vi "ScanIfSufficientPlaceHostDMA.vi"(8 "error in (no error)":errorcluster, 9 "Samples per Write":u32=1024000 format="%.3p", 10 "HSS Resource reference":refnum<k20>, 11 "TDMS controls in":T1[](array[typedef])) -> (0 "error out":errorcluster, 1 "Enough Space":bool, 2 "HSS Resource reference out":refnum<k20>, 3 "TDMS controls out":T1[](array[typedef]))   [LabVIEW 2018]
uses:
  TypeDefs/TDMS read.ctl
  <vilib>/Utility/error.llb/Error Cluster From Error Code.vi
  <vilib>/rvi/errors/niLvFpgaAdjustHostInterfaceError.vi
  <vilib>/rvi/interface/nirviMethod/nirviMethod.xnode
  <vilib>/FPGAPlugInAG/Dynamic/niLvFpga_AcquireWriteRegionFifo_Dynamic.vi
  <vilib>/rvi/errors/niLvFpgaMergeErrorWithErrorCode.vi
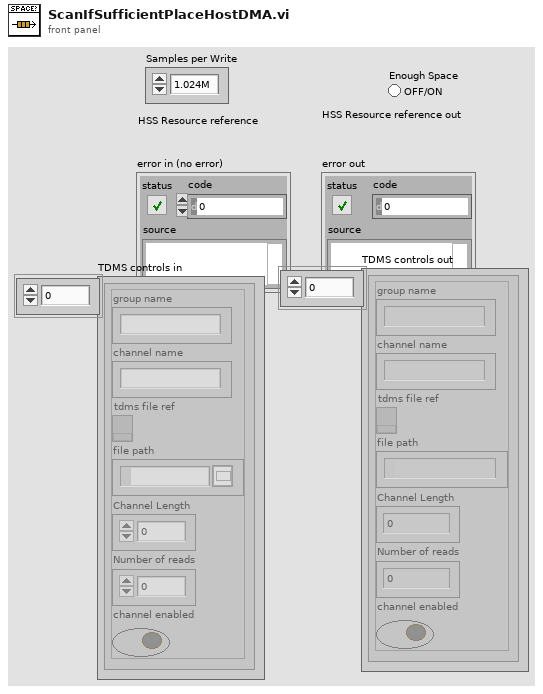
[diagram p1: front panel]
types:
  T1 = typedef "TDMS read.ctl" = cluster{"group name":string, "channel name":string, "tdms file ref":refnum<k34>, "file path":path, "Channel Length":i64, "Number of reads":i64, "channel enabled":bool}
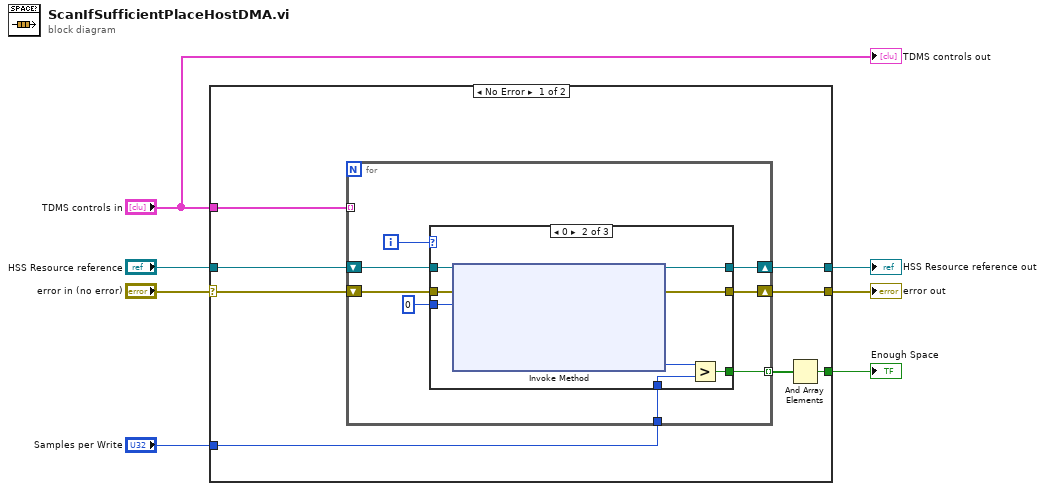
[diagram p0: block diagram]
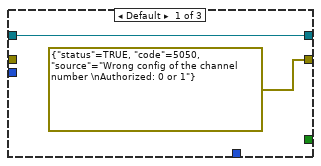
[diagram p2: hidden frame]
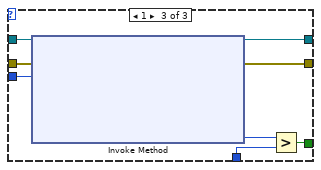
[diagram p3: hidden frame]
diagram:
  n1 = case shown="No Error" "error in (no error)" {
    selector: "error in (no error)" -> [w14 w43]
    tunnel: [w15 w43] -> w7
    tunnel: "Samples per Write" -> [w13 _]
    tunnel: [w11 _] -> w4
    tunnel: "HSS Resource reference" -> [w10 w42]
    tunnel: [w9 w42] -> w2
    tunnel: "TDMS controls in" -> [w8 _]
    frame No Error {
      n2 = for {
        shift-right: [w23] -> w15
        shift-left: w14 -> [w22]
        shift-right: [w21] -> w9
        shift-left: w10 -> [w20]
        tunnel: w13 -> [w18]
        tunnel: [w17] -> w12 mode=indexing
        tunnel: w8 -> [_] mode=indexing
        i -> [w16]
        n3 = case shown="0" w16 {
          tunnel: [errorcluster {"status"=TRUE, "code"=5050, "source"="Wrong config of the channel number \nAuthorized: 0 or 1"} ("error constant") w33 w41] -> w23
          tunnel: w22 -> [_ w32 w40]
          tunnel: [w25 w31 w39] -> w21
          tunnel: w20 -> [w25 w30 w38]
          tunnel: u32 0 ("Number of Elements") -> [_ w29 w37]
          tunnel: w18 -> [_ w27 w35]
          tunnel: [_ w26 w34] -> w17
          frame Default {
          }
          frame 0 {
            n4 = xnode "Invoke Method"("FPGA VI Reference In"=w30, "error in"=w32, "Number of Elements"=w29) -> ("FPGA VI Reference Out"=w31:refnum<k20>, "error out"=w33:errorcluster, "Empty Elements Remaining"=w28:u32)  [unwired: 1 in, 2 out]
            n5 = Greater?(x=w28, y=w27) -> (0:w26:bool)
          }
          frame 1 {
            n6 = xnode "Invoke Method"("FPGA VI Reference In"=w38, "error in"=w40, "Number of Elements"=w37) -> ("FPGA VI Reference Out"=w39:refnum<k20>, "error out"=w41:errorcluster, "Empty Elements Remaining"=w36:u32)  [unwired: 1 in, 2 out]
            n7 = Greater?(x=w36, y=w35) -> (0:w34:bool)
          }
        }
      }
      n8 = And Array Elements(Boolean array=w12) -> (logical AND=w11:bool)
    }
    frame Error {
    }
  }
  "error out" <- w7
  "Enough Space" <- w4
  "HSS Resource reference out" <- w2
  "TDMS controls out" <- "TDMS controls in"
